vi "FPGA Dynamic Ref PoC 2.vi"() -> ()   [LabVIEW 2025]
uses:
  <vilib>/userDefined/Silver/nirio_resource_slv.ctl
  <vilib>/FPGAPlugInAG/Dynamic/niLvFpga_Close_Dynamic.vi
  <vilib>/rvi/interface/nirviCloseFPGA/nirviCloseFPGA.xnode
  <instrlib>/FlexRIO/API/Host/v1/NI FlexRIO API v1.lvlib
panel:
  in  "Run When Loaded 2":bool
  in  "Run When Loaded":bool
  out "i 2":i32
  out "i":i32
  in  "Close 2":bool
  in  "Init 2":bool
  in  "stop 2":bool
  out "error out 2":errorcluster
  in  "Close":bool
  in  "Init":bool
  in  "stop":bool
  out "error out":errorcluster
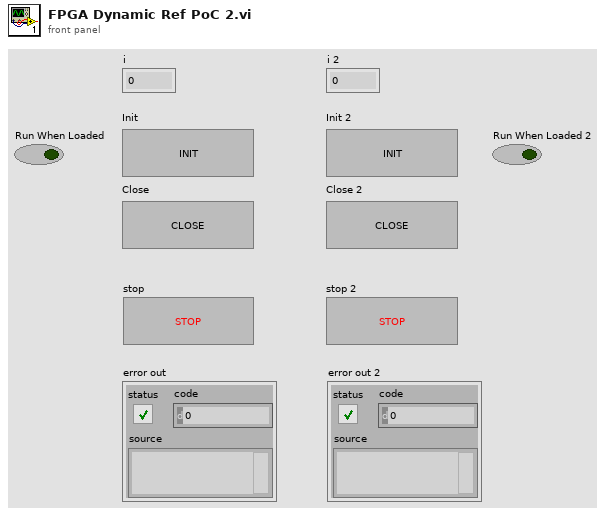
[diagram p1: front panel]
types:
  T1 = typedef "nirio_resource_slv.ctl" = tag
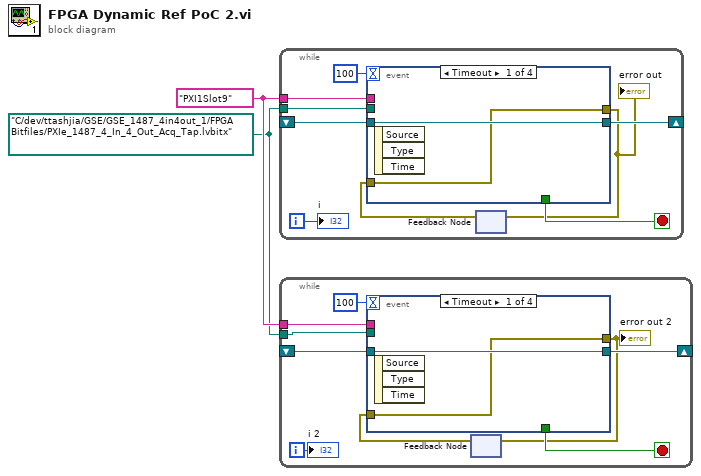
[diagram p0: block diagram]
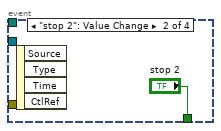
[diagram p2: hidden frame]
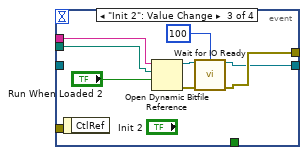
[diagram p3: hidden frame]
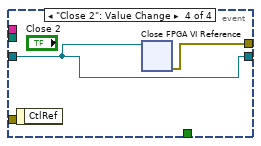
[diagram p4: hidden frame]
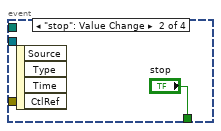
[diagram p5: hidden frame]
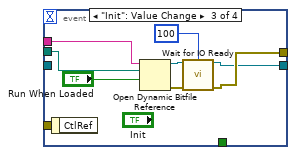
[diagram p6: hidden frame]
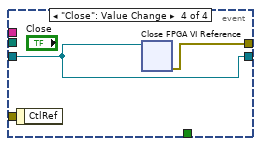
[diagram p7: hidden frame]
diagram:
  w1 = path "C:/dev/ttashjia/GSE/GSE_1487_4in4out_1/FPGA Bitfiles/PXIe_1487_4_In_4_Out_Acq_Tap.lvbitx" ("Bitfile path")
  w2 = T1 "PXI1Slot9" ("RIO Device")
  n1 = while {
    shift-right: [w10] -> _
    shift-left: _ -> [w9]
    tunnel: w2 -> [w8]
    tunnel: w1 -> [w7]
    i -> [w6]
    stop <- w11 stop-if-true
    n2 = feedback #1() -> (w4:errorcluster)  [unwired: 1 in]
    n3 = event shown="[0] Timeout" {
      selector: _ -> [_ _ _ _]
      dyn-events: _ -> [_ _ _ _]
      timeout: 100 -> [_ _ _ _]
      tunnel: [_ "stop" _ _] -> w11
      tunnel: [w12 _ w19 w24] -> w3
      tunnel: [w13 _ w18 w23] -> w10
      tunnel: w9 -> [w13 _ _ w23]
      tunnel: w8 -> [_ _ w17 _]
      tunnel: w7 -> [_ _ w16 _]
      tunnel: w4 -> [w12 _ _ _]
      event Timeout {
        n4 = event-data() -> ()  [unwired: 1 in, 3 out]
      }
      event "stop": Value Change {
        n5 = event-data() -> ()  [unwired: 1 in, 4 out]
      }
      event "Init": Value Change {
        n6 = event-data() -> ()  [unwired: 1 in, 1 out]
        n7 = Open Dynamic Bitfile Reference(0:w17, 1:w16, 2:"Run When Loaded") -> (5:w20:refnum<k20>, 8:w21:errorcluster)  [unwired: 2 in]
        n8 = call <instrlib>:"Wait for IO Ready.vi"("fpga interface in"=w20, "timeout"=100, "error in"=w21) -> ("fpga interface out"=w18:refnum<k20>, "error out"=w19:errorcluster)  [unwired: 9 in, 2 out]
      }
      event "Close": Value Change {
        n9 = event-data() -> ()  [unwired: 1 in, 1 out]
        n10 = xnode ("Close FPGA VI Reference")("FPGA VI Reference In"=w23) -> ("error out"=w24:errorcluster)  [unwired: 1 in]
      }
    }
    "error out" <- w3
    n11 = feedback-in #1(w3) -> ()
    "i" <- w6
  }
  n12 = while {
    shift-right: [w32] -> _
    shift-left: _ -> [w31]
    tunnel: w2 -> [w30]
    tunnel: w1 -> [w29]
    i -> [w28]
    stop <- w33 stop-if-true
    n13 = feedback #2() -> (w25:errorcluster)  [unwired: 1 in]
    n14 = event shown="[0] Timeout" {
      selector: _ -> [_ _ _ _]
      dyn-events: _ -> [_ _ _ _]
      timeout: 100 -> [_ _ _ _]
      tunnel: [_ "stop 2" _ _] -> w33
      tunnel: [w34 _ w41 w46] -> w26
      tunnel: [w35 _ w40 w45] -> w32
      tunnel: w31 -> [w35 _ _ w45]
      tunnel: w30 -> [_ _ w39 _]
      tunnel: w29 -> [_ _ w38 _]
      tunnel: w25 -> [w34 _ _ _]
      event Timeout {
        n15 = event-data() -> ()  [unwired: 1 in, 3 out]
      }
      event "stop 2": Value Change {
        n16 = event-data() -> ()  [unwired: 1 in, 4 out]
      }
      event "Init 2": Value Change {
        n17 = event-data() -> ()  [unwired: 1 in, 1 out]
        n18 = Open Dynamic Bitfile Reference(0:w39, 1:w38, 2:"Run When Loaded 2") -> (5:w42:refnum<k20>, 8:w43:errorcluster)  [unwired: 2 in]
        n19 = call <instrlib>:"Wait for IO Ready.vi"("fpga interface in"=w42, "timeout"=100, "error in"=w43) -> ("fpga interface out"=w40:refnum<k20>, "error out"=w41:errorcluster)  [unwired: 9 in, 2 out]
      }
      event "Close 2": Value Change {
        n20 = event-data() -> ()  [unwired: 1 in, 1 out]
        n21 = xnode ("Close FPGA VI Reference")("FPGA VI Reference In"=w45) -> ("error out"=w46:errorcluster)  [unwired: 1 in]
      }
    }
    "error out 2" <- w26
    n22 = feedback-in #2(w26) -> ()
    "i 2" <- w28
  }
